vi "HFRR ADV v019 new software.vi"() -> ()   [LabVIEW 2025] (continued)
        n324 = event-data() -> ()  [unwired: 1 in, 6 out]
        n325 = Unbundle By Name("Password 3") -> ("Service Password"=w413:string)
        n326 = call <vilib>:"Trim Whitespace.vi"("string"=w413) -> ("trimmed string"=w411:string)  [unwired: 1 in]
        n327 = Equal?(x=w411, y="Service@123") -> (x = y?=w412:bool)
        n328 = case shown="False" w412 {
          selector: w412 -> [w417 w419]
          frame False {
            n329 = local write "Service Password enable"(w417) -> ()
            n330 = property on="Service Password Log" class="Str"("Visible"=TRUE) -> ()  [unwired: 2 in, 2 out]
            n331 = property on="Tab Control 5" class="TabCtl (strict)"("Tabs Visible?"=TRUE ("Page Labels Display Visible?")) -> ()  [unwired: 2 in, 2 out]
          }
          frame True {
            n332 = property on="Service Password Log" class="Str"("Visible"=FALSE) -> ()  [unwired: 2 in, 2 out]
            "Service Password enable" <- w419
          }
        }
      }
      event "Sign In": Value Change {
        w421 = FALSE ("Visible")
        n333 = event-data() -> ()  [unwired: 1 in, 6 out]
        n334 = property on="About" class="Clust (strict)"("Visible"=w421) -> ()  [unwired: 2 in, 2 out]
        n335 = property on="Password 3" class="Clust (strict)"("Visible"=w421) -> ()  [unwired: 2 in, 2 out]
        n336 = property on="Service Password Log" class="Str"("Visible"=FALSE) -> ()  [unwired: 2 in, 2 out]
      }
      event "Info": Value Change {
        n337 = event-data() -> ()  [unwired: 1 in, 6 out]
        n338 = local read "Info"() -> (w423:bool)
        n339 = case shown="False" w423 {
          frame False {
            n340 = property on="About" class="Clust (strict)"("Visible"=FALSE) -> ()  [unwired: 2 in, 2 out]
          }
          frame True {
            n341 = property on="About" class="Clust (strict)"("Visible"=TRUE) -> ()  [unwired: 2 in, 2 out]
          }
        }
      }
      event "Calibration": Value Change {
        n342 = event-data() -> ()  [unwired: 1 in, 6 out]
        n343 = local read "Calibration"() -> (w427:bool)
        n344 = case shown="False" w427 {
          frame False {
            n345 = property on="Calibration 2" class="TabCtl (strict)"("Visible"=FALSE) -> ()  [unwired: 2 in, 2 out]
            n346 = local write "Cal Password"("" ("Cal Password")) -> ()
          }
          frame True {
            n347 = property on="Calibration 2" class="TabCtl (strict)"("Visible"=TRUE) -> ()  [unwired: 2 in, 2 out]
            n348 = local write "Cal Password"("" ("Cal Password")) -> ()
          }
        }
        n349 = property on="Wrong Password" class="Str"("Visible"=FALSE) -> ()  [unwired: 2 in, 2 out]
      }
      event "Cal Password": Value Change {
        n350 = event-data() -> ()  [unwired: 1 in, 6 out]
        n351 = local read "Cal Password"() -> (w435:string)
        n352 = call <vilib>:"Trim Whitespace.vi"("string"=w435) -> ("trimmed string"=w434:string)  [unwired: 1 in]
        n353 = Equal?(x=w434, y="Cal@321") -> (x = y?=w432:bool)
        n354 = case shown="True" w432 {
          frame False {
            n355 = property on="Wrong Password" class="Str"("Visible"=TRUE) -> ()  [unwired: 2 in, 2 out]
          }
          frame True {
            n356 = property on="Wrong Password" class="Str"("Visible"=FALSE) -> ()  [unwired: 2 in, 2 out]
            n357 = local write "Main Tab"(T2."About" ("Main Tab")) -> ()
            n358 = local write "Cal Password"("" ("Cal Password")) -> ()
            n359 = local write "Main Dashboard Buttons"(T1."About" ("Main Dashboard Buttons")) -> ()
            n360 = local write "Tab Control 5"(T12."Temperature Calibration" ("Tab Control 5")) -> ()
            n361 = property on="Calibration 2" class="TabCtl (strict)"("Visible"=FALSE) -> ()  [unwired: 2 in, 2 out]
            n362 = property on="Tab Control 5" class="TabCtl (strict)"("Tabs Visible?"=FALSE ("Page Labels Display Visible?")) -> ()  [unwired: 2 in, 2 out]
            n363 = local write "Calibration"(FALSE ("Calibration")) -> ()
          }
        }
      }
      event "Calibration Selection": Value Change {
        n364 = event-data() -> ()  [unwired: 1 in, 6 out]
        n365 = local read "Calibration Selection"() -> (w446:T8)
        n366 = case shown="\"Stroke Calibration\"" w446 {
          tunnel: [T7."Stroke" ("Main Calibration Tab") T7."Friction" ("Main Calibration Tab") T7."Main" ("Main Calibration Tab") T7."Temperature" ("Main Calibration Tab")] -> w445
          frame "Stroke Calibration" {
          }
          frame "Friction Force Calibration" {
          }
          frame Default {
          }
          frame "Temperature Calibration" {
          }
        }
        n367 = local write "Main Calibration Tab"(w445) -> ()
      }
      event "Back Stroke": Value Change {
        n368 = event-data() -> ()  [unwired: 1 in, 6 out]
        n369 = local write "Main Stroke Tab"(T9."Step 1" ("Main Stroke Tab")) -> ()
        n370 = local write "Main Calibration Tab"(T7."Main" ("Main Calibration Tab")) -> ()
        n371 = local write "Back Stroke"(FALSE ("Back Stroke")) -> ()
      }
      event "Step 2 Back": Value Change {
        n372 = event-data() -> ()  [unwired: 1 in, 6 out]
        n373 = local write "Main Stroke Tab"(T9."Step 1" ("Main Stroke Tab")) -> ()
        n374 = local write "Step 2 Back"(FALSE ("Back Stroke")) -> ()
      }
      event "Step 3 Back": Value Change {
        n375 = event-data() -> ()  [unwired: 1 in, 6 out]
        n376 = local write "Main Stroke Tab"(T9."Step 2" ("Main Stroke Tab")) -> ()
        n377 = local write "Step 3 Back"(FALSE ("Back Stroke")) -> ()
      }
      event "Step 4 Back": Value Change {
        n378 = event-data() -> ()  [unwired: 1 in, 6 out]
        n379 = local write "Main Stroke Tab"(T9."Step 3" ("Main Stroke Tab")) -> ()
        n380 = local write "Step 4 Back"(FALSE ("Back Stroke")) -> ()
      }
      event "Step 5 Back": Value Change {
        n381 = event-data() -> ()  [unwired: 1 in, 6 out]
        n382 = local write "Main Stroke Tab"(T9."Step 4" ("Main Stroke Tab")) -> ()
        n383 = local write "Step 5 Back"(FALSE ("Back Stroke")) -> ()
      }
      event "Step 6 Back": Value Change {
        n384 = event-data() -> ()  [unwired: 1 in, 6 out]
        n385 = local write "Main Stroke Tab"(T9."Step 5" ("Main Stroke Tab")) -> ()
        n386 = local write "Step 6 Back"(FALSE ("Back Stroke")) -> ()
      }
      event "Back Stroke step 7": Value Change {
        n387 = event-data() -> ()  [unwired: 1 in, 6 out]
        n388 = local write "Main Stroke Tab"(T9."Step 6" ("Main Stroke Tab")) -> ()
        n389 = local write "Back Stroke step 7"(FALSE ("Back Stroke")) -> ()
      }
      event "Back Stroke step 8": Value Change {
        n390 = event-data() -> ()  [unwired: 1 in, 6 out]
        n391 = local write "Main Stroke Tab"(T9."Step 7" ("Main Stroke Tab")) -> ()
        n392 = local write "Back Stroke step 8"(FALSE ("Back Stroke")) -> ()
      }
      event "Back Stroke 8": Value Change {
        n393 = event-data() -> ()  [unwired: 1 in, 6 out]
        n394 = local write "MOVE CARRIAGE TO"(0.2 ("MOVE CARRIAGE TO")) -> ()
        n395 = local write "Main Stroke Tab"(T9."Step 1" ("Main Stroke Tab")) -> ()
        n396 = local write "Back Stroke 8"(FALSE ("Back Stroke 8")) -> ()
      }
      event "Continue Stroke": Value Change {
        n397 = event-data() -> ()  [unwired: 1 in, 6 out]
        n398 = local write "Main Stroke Tab"(T9."Step 2" ("Main Stroke Tab")) -> ()
        n399 = local write "Continue Stroke"(FALSE ("Continue Stroke")) -> ()
      }
      event "Continue Stroke step 2": Value Change {
        n400 = event-data() -> ()  [unwired: 1 in, 6 out]
        n401 = local write "Main Stroke Tab"(T9."Step 3" ("Main Stroke Tab")) -> ()
        n402 = local write "Continue Stroke step 2"(FALSE ("Continue Stroke")) -> ()
      }
      event "Continue Stroke step 3": Value Change {
        n403 = event-data() -> ()  [unwired: 1 in, 6 out]
        n404 = local write "Main Stroke Tab"(T9."Step 4" ("Main Stroke Tab")) -> ()
        n405 = local write "Continue Stroke step 3"(FALSE ("Continue Stroke")) -> ()
      }
      event "Continue Stroke step 4": Value Change {
        n406 = event-data() -> ()  [unwired: 1 in, 6 out]
        n407 = local write "Main Stroke Tab"(T9."Step 5" ("Main Stroke Tab")) -> ()
        n408 = local write "Continue Stroke step 4"(FALSE ("Continue Stroke")) -> ()
      }
      event "Continue Stroke step 5": Value Change {
        n409 = event-data() -> ()  [unwired: 1 in, 6 out]
        n410 = local write "Main Stroke Tab"(T9."Step 6" ("Main Stroke Tab")) -> ()
        n411 = local write "Continue Stroke step 5"(FALSE ("Continue Stroke")) -> ()
      }
      event "Continue Stroke step 6": Value Change {
        n412 = event-data() -> ()  [unwired: 1 in, 6 out]
        n413 = local write "Main Stroke Tab"(T9."Step 7" ("Main Stroke Tab")) -> ()
        n414 = local write "Continue Stroke step 6"(FALSE ("Continue Stroke")) -> ()
      }
      event "Continue Stroke step 7": Value Change {
        w485 = FALSE ("0.2mm")
        n415 = event-data() -> ()  [unwired: 1 in, 6 out]
        n416 = local write "0.4 mm"(w485) -> ()
        n417 = local write "0.6 mm"(w485) -> ()
        n418 = local write "1.0 mm"(w485) -> ()
        n419 = local write "1.2 mm"(w485) -> ()
        n420 = local write "0.2 2"(w485) -> ()
        n421 = local write "0.4 2"(w485) -> ()
        n422 = local write "0.6 2"(w485) -> ()
        n423 = local write "0.8 2"(w485) -> ()
        n424 = local write "1.0 2"(w485) -> ()
        n425 = local write "1.2"(w485) -> ()
        n426 = local write "0.2mm"(w485) -> ()
        n427 = local write "0.8mm"(w485) -> ()
        n428 = local write "Main Stroke Tab"(T9."Step 8" ("Main Stroke Tab")) -> ()
        n429 = local write "Continue Stroke step 7"(FALSE ("Continue Stroke")) -> ()
        n430 = local write "Stroke Test Complete"(T10."Test Progress" ("Stroke Test Complete")) -> ()
        "Position Measurment Temp" <- 0.0 ("Position Measurment Temp")
        "Calibration Tare" <- TRUE ("Calibration Tare")
        "MOVE CARRIAGE TO" <- 0.2 ("MOVE CARRIAGE TO")
      }
      event "Continue Stroke step 8": Value Change {
        n431 = event-data() -> ()  [unwired: 1 in, 6 out]
        n432 = local read "LVDT STROKE  Calibration"() -> (w490:dbl)
        n433 = local read "Position Measurment Temp"() -> (w491:dbl)
        n434 = case shown="4" w491 {
          selector: w491 -> [w496 w501 w506 w511 w516 w520 w523 w524]
          tunnel: w490 -> [w492 w497 w502 w507 w512 w517 _ _]
          frame 0, Default {
            w494 = TRUE ("0.2mm")
            n435 = Increment(x=w496) -> (x+1=w495:i32)
            n436 = local write "Position Measurment Temp"(w495) -> ()
            n437 = local write "0.2mm"(w494) -> ()
            n438 = local write "0.2 2"(w494) -> ()
            n439 = local write "MOVE CARRIAGE TO"(0.4 ("MOVE CARRIAGE TO")) -> ()
            "Calibration 0.2" <- w492
          }
          frame 1 {
            w499 = TRUE ("0.4 mm")
            n440 = Increment(x=w501) -> (x+1=w500:i32)
            n441 = local write "Calibration 0.4"(w497) -> ()
            n442 = local write "Position Measurment Temp"(w500) -> ()
            n443 = local write "0.4 mm"(w499) -> ()
            n444 = local write "MOVE CARRIAGE TO"(0.6 ("MOVE CARRIAGE TO")) -> ()
            n445 = local write "0.4 2"(w499) -> ()
          }
          frame 2 {
            w504 = TRUE ("0.6 mm")
            n446 = Increment(x=w506) -> (x+1=w505:i32)
            n447 = local write "Calibration 0.6"(w502) -> ()
            n448 = local write "Position Measurment Temp"(w505) -> ()
            n449 = local write "0.6 2"(w504) -> ()
            n450 = local write "0.6 mm"(w504) -> ()
            n451 = local write "MOVE CARRIAGE TO"(0.8 ("MOVE CARRIAGE TO")) -> ()
          }
          frame 3 {
            w508 = TRUE ("0.6 mm")
            n452 = Increment(x=w511) -> (x+1=w510:i32)
            n453 = local write "Position Measurment Temp"(w510) -> ()
            n454 = local write "MOVE CARRIAGE TO"(1.0 ("MOVE CARRIAGE TO")) -> ()
            n455 = local write "0.8mm"(w508) -> ()
            n456 = local write "0.8 2"(w508) -> ()
            "Calibration 0.8" <- w507
          }
          frame 4 {
            w513 = TRUE ("0.6 mm")
            n457 = Increment(x=w516) -> (x+1=w515:i32)
            n458 = local write "Position Measurment Temp"(w515) -> ()
            n459 = local write "MOVE CARRIAGE TO"(1.2 ("MOVE CARRIAGE TO")) -> ()
            n460 = local write "1.0 mm"(w513) -> ()
            n461 = local write "1.0 2"(w513) -> ()
            "Calibration 1.0" <- w512
          }
          frame 5 {
            w518 = TRUE ("0.6 mm")
            n462 = Increment(x=w520) -> (x+1=w519:i32)
            n463 = local write "Position Measurment Temp"(w519) -> ()
            n464 = local write "1.2 mm"(w518) -> ()
            n465 = local write "1.2"(w518) -> ()
            "Calibration 1.2" <- w517
          }
          frame 6 {
            n466 = Increment(x=w523) -> (x+1=w522:i32)
            n467 = local write "Position Measurment Temp"(w522) -> ()
            n468 = local write "Stroke Test Complete"(T10."Stroke Points Completed" ("Stroke Test Complete")) -> ()
          }
          frame 7 {
            n469 = stacked-sequence {
              tunnel: w524 -> [w525 _ _]
              frame #0 {
                n470 = Increment(x=w525) -> (x+1=w526:i32)
                n471 = local write "Main Stroke Tab"(T9."Step 9" ("Main Stroke Tab")) -> ()
                n472 = local write "Position Measurment Temp"(w526) -> ()
                n473 = Insert Into Array(array=dbl[] [], new element #1=0.2 ("new element/subarray"), new element #2=0.4 ("new element/subarray"), new element #3=0.6 ("new element/subarray"), new element #4=0.8 ("new element/subarray"), new element #5=1.0 ("new element/subarray"), new element #6=1.2 ("new element/subarray")) -> (→"1D stroke":dbl[])  [unwired: 1 in]
                n474 = local read "Calibration 0.2"() -> (w533:dbl)
                n475 = local read "Calibration 0.4"() -> (w532:dbl)
                n476 = local read "Calibration 0.6"() -> (w531:dbl)
                n477 = local read "Calibration 0.8"() -> (w530:dbl)
                n478 = local read "Calibration 1.0"() -> (w529:dbl)
                n479 = local read "Calibration 1.2"() -> (w528:dbl)
                n480 = Insert Into Array(array=dbl[] [], new element #1=w533, new element #2=w532, new element #3=w531, new element #4=w530, new element #5=w529, new element #6=w528) -> (→"Calibrated Voltage Value":dbl[])  [unwired: 1 in]
              }
              frame #1 {
                n481 = local read "Calibrated Voltage Value"() -> (w545:dbl[])
                n482 = local read "1D stroke"() -> (w546:dbl[])
                n483 = for {
                  tunnel: [w549] -> w544 mode=indexing
                  tunnel: w546 -> [w548] mode=indexing
                  tunnel: w545 -> [w547] mode=indexing
                  n484 = formula code="if (stroke == 0.2) {\n    status = (voltage >= 0.0961 && voltage <= 0.4961) ? 1 : 0;\n} else if (stroke == 0.4) {\n    status = (voltage >= 0.3425 && voltage <= 0.7425) ? 1 : 0;\n} else if (stroke == 0.6) {\n    status = (voltage >= 0.5370 && voltage <= 0.9370) ? 1 : 0;\n} else if (stroke == 0.8) {\n    status = (voltage >= 0.6640 && voltage <= 1.0640) ? 1 : 0;\n} else if (stroke == 1.0) {\n    status = (voltage >= 0.9000 && voltage <= 1.1000) ? 1 : 0;\n} else if (stroke == 1.2) {\n    status = (voltage >= 0.9278 && voltage <= 1.3278) ? 1 : 0;\n} else {\n    status = 0; // Fails if an invalid stroke value is supplied\n}"("stroke"=w548, "voltage"=w547) -> ("status"=w549:dbl)
                }
                "Status" <- w544
              }
              frame #2 {
                w556 = 1.0
                n485 = local read "Status"() -> (w563:dbl[])
                n486 = Index Array(array=w563) -> (element #1=w562:dbl, element #2=w561:dbl, element #3=w560:dbl, element #4=w559:dbl, element #5=w558:dbl, element #6=w557:dbl)  [unwired: 6 in]
                n487 = Equal?(x=w561, y=w556) -> (x = y?=w554:bool)
                n488 = Equal?(x=w560, y=w556) -> (x = y?=w553:bool)
                n489 = Equal?(x=w559, y=w556) -> (x = y?=w552:bool)
                n490 = Equal?(x=w558, y=w556) -> (x = y?=w551:bool)
                n491 = Equal?(x=w557, y=w556) -> (x = y?=w550:bool)
                n492 = Equal?(x=w562, y=w556) -> (x = y?=w555:bool)
                n493 = case shown="True" w555 {
                  selector: w555 -> [w574 w575]
                  frame True {
                    n494 = local write "Point 1 - 0.2 mm"(w574) -> ()
                    n495 = property on="Point 1 - 0.2 mm" class="Bool"("Caption.Visible"=w574) -> ()  [unwired: 2 in, 2 out]
                  }
                  frame False {
                    n496 = local write "Point 1 - 0.2 mm"(w575) -> ()
                    n497 = property on="Point 1 - 0.2 mm" class="Bool"("Caption.Visible"=w575) -> ()  [unwired: 2 in, 2 out]
                  }
                }
                n498 = case shown="True" w554 {
                  selector: w554 -> [w572 w573]
                  frame True {
                    n499 = local write "Point 2 - 0.4 mm"(w572) -> ()
                    n500 = property on="Point 2 - 0.4 mm" class="Bool"("Caption.Visible"=w572) -> ()  [unwired: 2 in, 2 out]
                  }
                  frame False {
                    n501 = local write "Point 2 - 0.4 mm"(w573) -> ()
                    n502 = property on="Point 2 - 0.4 mm" class="Bool"("Caption.Visible"=w573) -> ()  [unwired: 2 in, 2 out]
                  }
                }
                n503 = case shown="True" w551 {
                  selector: w551 -> [w566 w567]
                  frame True {
                    n504 = local write "Point 5 - 1.0 mm"(w566) -> ()
                    n505 = property on="Point 5 - 1.0 mm" class="Bool"("Caption.Visible"=w566) -> ()  [unwired: 2 in, 2 out]
                  }
                  frame False {
                    n506 = local write "Point 5 - 1.0 mm"(w567) -> ()
                    n507 = property on="Point 5 - 1.0 mm" class="Bool"("Caption.Visible"=w567) -> ()  [unwired: 2 in, 2 out]
                  }
                }
                n508 = case shown="True" w553 {
                  selector: w553 -> [w570 w571]
                  frame True {
                    n509 = local write "Point 3 - 0.6 mm"(w570) -> ()
                    n510 = property on="Point 3 - 0.6 mm" class="Bool"("Caption.Visible"=w570) -> ()  [unwired: 2 in, 2 out]
                  }
                  frame False {
                    n511 = local write "Point 3 - 0.6 mm"(w571) -> ()
                    n512 = property on="Point 3 - 0.6 mm" class="Bool"("Caption.Visible"=w571) -> ()  [unwired: 2 in, 2 out]
                  }
                }
                n513 = case shown="True" w552 {
                  selector: w552 -> [w568 w569]
                  frame True {
                    n514 = local write "Point 4 - 0.8 mm"(w568) -> ()
                    n515 = property on="Point 4 - 0.8 mm" class="Bool"("Caption.Visible"=w568) -> ()  [unwired: 2 in, 2 out]
                  }
                  frame False {
                    n516 = local write "Point 4 - 0.8 mm"(w569) -> ()
                    n517 = property on="Point 4 - 0.8 mm" class="Bool"("Caption.Visible"=w569) -> ()  [unwired: 2 in, 2 out]
                  }
                }
                n518 = case shown="True" w550 {
                  selector: w550 -> [w564 w565]
                  frame True {
                    n519 = local write "Point 6 - 1.2 mm"(w564) -> ()
                    n520 = property on="Point 6 - 1.2 mm" class="Bool"("Caption.Visible"=w564) -> ()  [unwired: 2 in, 2 out]
                  }
                  frame False {
                    n521 = local write "Point 6 - 1.2 mm"(w565) -> ()
                    n522 = property on="Point 6 - 1.2 mm" class="Bool"("Caption.Visible"=w565) -> ()  [unwired: 2 in, 2 out]
                  }
                }
              }
            }
          }
        }
      }
      event "TEMPERATURE STEP Back 1", "TEMPERATURE STEP Back air Temp": Value Change {
        n523 = event-data() -> ()  [unwired: 1 in, 6 out]
        n524 = stacked-sequence {
          frame #0 {
            n525 = local write "Main Calibration Tab"(T7."Main" ("Main Calibration Tab")) -> ()
          }
          frame #1 {
            n526 = Wait (ms)(milliseconds to wait=u32 1000) -> ()  [unwired: 1 out]
          }
          frame #2 {
            n527 = local write "Command"("CAL;END" ("Command")) -> ()
          }
          frame #3 {
            n528 = Wait (ms)(milliseconds to wait=u32 2000) -> ()  [unwired: 1 out]
          }
          frame #4 {
            n529 = local write "Command"("CAL;END" ("Command")) -> ()
          }
        }
      }
      event "Temperature Continue Step 1": Value Change {
        n530 = event-data() -> ()  [unwired: 1 in, 6 out]
        n531 = stacked-sequence {
          frame #0 {
            n532 = Wait (ms)(milliseconds to wait=u32 1500) -> ()  [unwired: 1 out]
          }
          frame #1 {
            n533 = local write "Command"("CAL;START" ("Command")) -> ()
          }
          frame #2 {
            n534 = Wait (ms)(milliseconds to wait=u32 1500) -> ()  [unwired: 1 out]
          }
          frame #3 {
            n535 = local write "Command"("CAL;START" ("Command")) -> ()
          }
          frame #4 {
            n536 = Wait (ms)(milliseconds to wait=u32 2000) -> ()  [unwired: 1 out]
          }
          frame #5 {
          }
          frame #6 {
            n537 = Wait (ms)(milliseconds to wait=u32 2000) -> ()  [unwired: 1 out]
          }
          frame #7 {
            # "CAL;A1;<true_T>"
            n538 = local write "Command"("CAL;A1;0" ("Command")) -> ()
          }
          frame #8 {
            n539 = local write "Tab Control 4"(T11."Step 2" ("Tab Control 4")) -> ()
          }
        }
      }
      event "Temperature Continue Step air Step 1": Value Change {
        n540 = event-data() -> ()  [unwired: 1 in, 6 out]
        n541 = stacked-sequence {
          frame #0 {
            n542 = Wait (ms)(milliseconds to wait=u32 1500) -> ()  [unwired: 1 out]
          }
          frame #1 {
            n543 = local write "Command"("CAL;START" ("Command")) -> ()
          }
          frame #2 {
            n544 = local write "Tab Control 4"(T11."Air Step 2" ("Tab Control 4")) -> ()
            n545 = Wait (ms)(milliseconds to wait=u32 1500) -> ()  [unwired: 1 out]
          }
          frame #3 {
            n546 = local write "Command"("CAL;START" ("Command")) -> ()
          }
          frame #4 {
            n547 = Wait (ms)(milliseconds to wait=u32 2000) -> ()  [unwired: 1 out]
          }
          frame #5 {
            # "CAL;A1;<true_T>"
            n548 = local write "Command"("CAL;A2;0" ("Command")) -> ()
          }
          frame #6 {
            n549 = Wait (ms)(milliseconds to wait=u32 2000) -> ()  [unwired: 1 out]
          }
          frame #7 {
            # "CAL;A1;<true_T>"
            n550 = local write "Command"("CAL;A1;0" ("Command")) -> ()
          }
        }
      }
      event "Temperature Selection": Value Change {
        n551 = event-data() -> ()  [unwired: 1 in, 6 out]
        n552 = local read "Temperature Selection"() -> (w598:enum32{"Air Temperature", "Sample Temperature"})
        n553 = case shown="\"Sample Temperature\"" w598 {
          frame "Air Temperature", Default {
            n554 = local write "Tab Control 4"(T11."Air Step 1" ("Tab Control 4")) -> ()
          }
          frame "Sample Temperature" {
            n555 = local write "Tab Control 4"(T11."Step 1" ("Tab Control 4")) -> ()
          }
        }
      }
      event "Temperature Continue Step 2": Value Change {
        n556 = event-data() -> ()  [unwired: 1 in, 6 out]
        n557 = stacked-sequence {
          frame #0 {
            n558 = stacked-sequence {
              frame #0 {
                n559 = Wait (ms)(milliseconds to wait=u32 1500) -> ()  [unwired: 1 out]
              }
              frame #1 {
                # "CAL;A1;<true_T>"
                n560 = local write "Command"("CAL;A1;0" ("Command")) -> ()
              }
              frame #2 {
                n561 = Wait (ms)(milliseconds to wait=u32 1500) -> ()  [unwired: 1 out]
              }
              frame #3 {
                # "CAL;A1;<true_T>"
                n562 = local write "Command"("CAL;A1;0" ("Command")) -> ()
              }
              frame #4 {
              }
            }
          }
          frame #1 {
            n563 = local write "Tab Control 4"(T11."Step 3" ("Tab Control 4")) -> ()
          }
        }
      }
      event "Temperature Continue Step 3": Value Change {
        n564 = event-data() -> ()  [unwired: 1 in, 6 out]
        n565 = stacked-sequence {
          frame #0 {
            n566 = stacked-sequence {
              frame #0 {
                n567 = Wait (ms)(milliseconds to wait=u32 1500) -> ()  [unwired: 1 out]
              }
              frame #1 {
              }
              frame #2 {
              }
              frame #3 {
                # "CAL;A1;<true_T>"
                n568 = local write "Command"("CAL;A1;60" ("Command")) -> ()
              }
              frame #4 {
                n569 = Wait (ms)(milliseconds to wait=u32 2000) -> ()  [unwired: 1 out]
              }
              frame #5 {
                # "CAL;A1;<true_T>"
                n570 = local write "Command"("CAL;A1;60" ("Command")) -> ()
              }
            }
          }
          frame #1 {
            n571 = Wait (ms)(milliseconds to wait=u32 1000) -> ()  [unwired: 1 out]
          }
          frame #2 {
            n572 = local write "Command"("CAL;SAVE" ("Command")) -> ()
          }
          frame #3 {
            n573 = Wait (ms)(milliseconds to wait=u32 1000) -> ()  [unwired: 1 out]
          }
          frame #4 {
            n574 = local write "Command"("CAL;SAVE" ("Command")) -> ()
          }
          frame #5 {
            n575 = Wait (ms)(milliseconds to wait=u32 1000) -> ()  [unwired: 1 out]
          }
          frame #6 {
            # "CAL;END"
            n576 = local write "Command"("CAL;END" ("Command")) -> ()
          }
          frame #7 {
            n577 = Wait (ms)(milliseconds to wait=u32 1000) -> ()  [unwired: 1 out]
          }
          frame #8 {
            # "CAL;END"
            n578 = local write "Command"("CAL;END" ("Command")) -> ()
          }
          frame #9 {
            n579 = local write "Main Calibration Tab"(T7."Temperature" ("Main Calibration Tab")) -> ()
            n580 = local write "Tab Control 4"(T11."Main" ("Tab Control 4")) -> ()
          }
        }
      }
      event "Back Stroke step main temperature": Value Change {
        n581 = event-data() -> ()  [unwired: 1 in, 6 out]
        n582 = stacked-sequence {
          frame #0 {
            n583 = Wait (ms)(milliseconds to wait=u32 1000) -> ()  [unwired: 1 out]
          }
          frame #1 {
            # "CAL;END"
            n584 = local write "Command"("CAL;END" ("Command")) -> ()
          }
          frame #2 {
            n585 = Wait (ms)(milliseconds to wait=u32 1000) -> ()  [unwired: 1 out]
          }
          frame #3 {
            # "CAL;END"
            n586 = local write "Command"("CAL;END" ("Command")) -> ()
          }
          frame #4 {
            n587 = local write "Main Calibration Tab"(T7."Temperature" ("Main Calibration Tab")) -> ()
            n588 = local write "Tab Control 4"(T11."Main" ("Tab Control 4")) -> ()
          }
        }
      }
      event "Quit": Value Change {
        n589 = event-data() -> ()  [unwired: 1 in, 6 out]
      }
    }
    n590 = Wait (ms)(milliseconds to wait=u32 100) -> ()  [unwired: 1 out]
  }
  n591 = while {
    stop <- w630 stop-if-true
    n592 = local read "Ambient Temperature"() -> (w628:dbl)
    n593 = local read "Sample Temperature"() -> (w627:dbl)
    n594 = local write "Temperature — Live (Set A: 60 °C)"(w627) -> ()
    n595 = local write "Temperature — Live (Set A: 60 °C)"(w627) -> ()
    n596 = local write "Temperature — Live (Set A: 0 °C)"(w628) -> ()
    n597 = local write "Sensor value"(w628) -> ()
    n598 = local write "Sensor value"(w627) -> ()
    n599 = local write "Temperature — Live (Set A: 60 °C)"(w628) -> ()
    n600 = local write "Sensor value"(w627) -> ()
    n601 = local write "Sensor value"(w628) -> ()
    n602 = Wait (ms)(milliseconds to wait=u32 200) -> ()  [unwired: 1 out]
    n603 = local read "Quit"() -> (w630:bool)
  }
  n604 = while {
    shift-right: [w632] -> _
    shift-left: "Enum - Selector" -> [w633]
    stop <- w634 stop-if-true
    # "Auto Start Logic Loop"
    n605 = case shown="\"Humidity & Temperature On\"" w633 {
      tunnel: [w637 w643 w670 w702 w732 Auto_Start_enum."Exit" ("Enum - Selector") Auto_Start_enum."Init" ("Enum - Selector")] -> w632
      frame "Init", Default {
        n606 = local read "Auto Start Test"() -> (w636:bool)
        n607 = Select(t=Auto_Start_enum."Humidity & Temperature On" ("Enum - Selector"), s=w636, f=Auto_Start_enum."Init") -> (s? t:f=w637:T15)
      }
      frame "Humidity & Temperature On" {
        n608 = stacked-sequence {
          tunnel: [_ _ _ _ _ _ Auto_Start_enum."Reach point" ("Enum - Selector")] -> w640
          frame #0 {
            w645 = T19."Disabled and Grayed Out" ("Disabled")
            w646 = TRUE ("Heater Button")
            n609 = property on="Humidity" class="Bool (strict)"("DisabledEnum"=w645) -> ()  [unwired: 2 in, 2 out]
            n610 = property on="Heater Button" class="Bool (strict)"("DisabledEnum"=w645) -> ()  [unwired: 2 in, 2 out]
            n611 = local write "Heater Button"(w646) -> ()
            n612 = local write "Humidity"(w646) -> ()
            n613 = property on="Heater Button" class="Bool (strict)"("Val(Sgnl)"=TRUE ("Value (Signaling)")) -> ()  [unwired: 2 in, 2 out]
          }
          frame #1 {
            n614 = Wait (ms)(milliseconds to wait=u32 3000) -> ()  [unwired: 1 out]
          }
          frame #2 {
            n615 = local read "Set Temp"() -> (w652:dbl)
            n616 = Number To Fractional String(number=w652, precision (6)=i16 2) -> (F-format string=w649:string)  [unwired: 2 in]
            n617 = Concatenate Strings("ST;" ("Command"), w649) -> (w650:string)
            n618 = local write "Command"(w650) -> ()
          }
          frame #3 {
            n619 = Wait (ms)(milliseconds to wait=u32 1500) -> ()  [unwired: 1 out]
          }
          frame #4 {
            (unwired) i16 2 ("precision (6)")
            n620 = local read "WriteHumidity 2"() -> (w654:string[])
            n621 = local read "Set Rh"() -> (w657:dbl)
            n622 = Number To Fractional String(number=w657) -> (F-format string=w658:string)  [unwired: 3 in]
            n623 = Concatenate Strings("M;" ("new element/subarray"), w658) -> (w659:string)
            n624 = local write "Command"("HE;1" ("Command")) -> ()
            n625 = Insert Into Array(array=w654, new element=w659) -> (w655:string[])  [unwired: 1 in]
            n626 = local write "WriteHumidity 2"(w655) -> ()
          }
          frame #5 {
            n627 = Wait (ms)(milliseconds to wait=u32 1500) -> ()  [unwired: 1 out]
          }
          frame #6 {
            w662 = TRUE ("Reach point temp")
            n628 = local write "Reach point Humidity"(w662) -> ()
            n629 = local write "Reach point temp"(w662) -> ()
          }
        }
        n630 = local read "Auto Start Test"() -> (w642:bool)
        n631 = Not(x=w642) -> (.not. x?=w641:bool)
        n632 = Select(t=Auto_Start_enum."close", s=w641, f=w640) -> (s? t:f=w643:T15)
      }
      frame "Reach point" {
        w671 = TRUE ("PAUSE")
        w679 = 1.0 ("y")
        w682 = 1.0 ("y")
        n633 = local read "Set Temp"() -> (w664:dbl)
        n634 = local read "Set Humidity:"() -> (w678:dbl)
        n635 = local read "Humidity ( %RH )"() -> (w683:dbl)
        n636 = Add(x=w664, y=w682) -> (x+y=w681:dbl)
        n637 = Subtract(x=w664, y=w682) -> (x-y=w680:dbl)
        n638 = Add(x=w678, y=w679) -> (x+y=w677:dbl)
        n639 = Subtract(x=w678, y=w679) -> (x-y=w676:dbl)
        n640 = local read "TEMP"() -> (w684:dbl)
        n641 = In Range and Coerce(upper limit=w677, x=w683, lower limit=w676) -> (In Range?=w665:bool)  [unwired: 1 out]
        n642 = In Range and Coerce(upper limit=w681, x=w684, lower limit=w680) -> (In Range?=w666:bool)  [unwired: 1 out]
        n643 = case shown="True" w665 {
          frame False {
          }
          frame True {
            n644 = case shown="True" "Reach point Humidity" {
              selector: "Reach point Humidity" -> [_ w690]
              frame False {
              }
              frame True {
                n645 = local read "EVENT LOG"() -> (w687:string)
                n646 = Not(x=w690) -> (.not. x?=w689:bool)
                n647 = local write "Reach point Humidity"(w689) -> ()
                n648 = call "Event Log.vi"("Content"="Target Humidity reached", "EVENT LOG"=w687) -> ("EVENT LOG"=w688:string)  [unwired: 8 in, 1 out]
                n649 = local write "EVENT LOG"(w688) -> ()
              }
            }
          }
        }
        n650 = case shown="True" w666 {
          frame False {
          }
          frame True {
            n651 = case shown="True" "Reach point temp" {
              selector: "Reach point temp" -> [_ w696]
              frame False {
              }
              frame True {
                n652 = local read "EVENT LOG"() -> (w693:string)
                n653 = Not(x=w696) -> (.not. x?=w695:bool)
                n654 = local write "Reach point temp"(w695) -> ()
                n655 = call "Event Log.vi"("Content"="Target Temperature reached", "EVENT LOG"=w693) -> ("EVENT LOG"=w694:string)  [unwired: 8 in, 1 out]
                n656 = local write "EVENT LOG"(w694) -> ()
              }
            }
          }
        }
        n657 = local read "Auto Start Test"() -> (w669:bool)
        n658 = And(x=w666, y=w665) -> (x .and. y?=w675:bool)
        n659 = Select(t=Auto_Start_enum."Maintain Stage" ("Enum - Selector"), s=w675, f=Auto_Start_enum."Reach point" ("Enum - Selector")) -> (s? t:f=w672:T15)
        n660 = Not(x=w669) -> (.not. x?=w668:bool)
        n661 = Select(t=Auto_Start_enum."close", s=w668, f=w672) -> (s? t:f=w670:T15)
        n662 = call "ELAPSED TIMER VI.vi"("RESET"=w671, "PAUSE"=w671) -> ()  [unwired: 7 in, 3 out]
      }
      frame "Maintain Stage" {
        w711 = 2.0 ("y")
        w710 = 1.0 ("y")
        # "Humidity and  temperatures Set Point  have been reached"
        n663 = local read "Set Temp"() -> (w697:dbl)
        n664 = local read "Set Humidity:"() -> (w714:dbl)
        n665 = local read "Humidity ( %RH )"() -> (w717:dbl)
        n666 = Add(x=w697, y=w710) -> (x+y=w716:dbl)
        n667 = Subtract(x=w697, y=w710) -> (x-y=w715:dbl)
        n668 = local read "TEMP"() -> (w718:dbl)
        n669 = Add(x=w714, y=w711) -> (x+y=w713:dbl)
        n670 = Subtract(x=w714, y=w711) -> (x-y=w712:dbl)
        n671 = In Range and Coerce(upper limit=w716, x=w718, lower limit=w715) -> (In Range?=w709:bool)  [unwired: 1 out]
        n672 = In Range and Coerce(upper limit=w713, x=w717, lower limit=w712) -> (In Range?=w708:bool)  [unwired: 1 out]
        n673 = And(x=w709, y=w708) -> (x .and. y?=w707:bool)
        n674 = Not(x=w707) -> (.not. x?=w706:bool)
        n675 = call "ELAPSED TIMER VI.vi"("TARGET"=60.0, "RESET"=w706, "PAUSE"=FALSE) -> ("ELAPSED INDICATION"=w703:bool)  [unwired: 6 in, 2 out]
        n676 = case shown="True" w703 {
          tunnel: w703 -> [_ w721]
          tunnel: [Auto_Start_enum."Maintain Stage" ("Enum - Selector") w720] -> w701
          frame False {
          }
          frame True {
            n677 = stacked-sequence {
              tunnel: w721 -> [_ _ _ _ _]
              tunnel: [_ _ _ _ Auto_Start_enum."Start Stage" ("Enum - Selector")] -> w720
              frame #0 {
                n678 = local read "EVENT LOG"() -> (w723:string)
                n679 = call "Event Log.vi"("Content"="Humidity and temperature set point has stabilized.", "EVENT LOG"=w723) -> ("EVENT LOG"=w724:string)  [unwired: 8 in, 1 out]
                n680 = local write "EVENT LOG"(w724) -> ()
              }
              frame #1 {
                n681 = Wait (ms)(milliseconds to wait=u32 100) -> ()  [unwired: 1 out]
              }
              frame #2 {
                n682 = local read "EVENT LOG"() -> (w727:string)
                n683 = call "Event Log.vi"("Content"="Auto Test Started", "EVENT LOG"=w727) -> ("EVENT LOG"=w728:string)  [unwired: 8 in, 1 out]
                n684 = local write "EVENT LOG"(w728) -> ()
              }
              frame #3 {
                w729 = TRUE ("RUN")
                n685 = local write "RUN"(w729) -> ()
                n686 = property on="Auto Start Temp" class="Bool (strict)"("Val(Sgnl)"=w729) -> ()  [unwired: 2 in, 2 out]
                "Auto Start Temp" <- w729
              }
              frame #4 {
              }
            }
          }
        }
        n687 = local read "Auto Start Test"() -> (w700:bool)
        n688 = Not(x=w700) -> (.not. x?=w699:bool)
        n689 = Select(t=Auto_Start_enum."close", s=w699, f=w701) -> (s? t:f=w702:T15)
      }
      frame "Start Stage" {
        w731 = TRUE ("PAUSE")
        n690 = local read "Auto Start Test"() -> (w736:bool)
        n691 = Not(x=w736) -> (.not. x?=w735:bool)
        n692 = Select(t=Auto_Start_enum."close" ("Enum - Selector"), s=w735, f=Auto_Start_enum."Start Stage" ("Enum - Selector")) -> (s? t:f=w732:T15)
        n693 = call "ELAPSED TIMER VI.vi"("RESET"=w731, "PAUSE"=w731) -> ()  [unwired: 7 in, 3 out]
      }
      frame "close" {
        w738 = FALSE ("Heater Button")
        n694 = local write "RUN"(w738) -> ()
        n695 = local write "Heater Button"(w738) -> ()
        n696 = local write "Humidity"(w738) -> ()
        n697 = local write "Auto Start Test"(w738) -> ()
        n698 = property on="Heater Button" class="Bool (strict)"("Val(Sgnl)"=FALSE ("Value (Signaling)")) -> ()  [unwired: 2 in, 2 out]
      }
      frame "Exit" {
      }
    }
    n699 = Wait (ms)(milliseconds to wait=u32 100) -> ()  [unwired: 1 out]
    n700 = local read "Quit"() -> (w634:bool)
  }
  n701 = property on="Service Password Log" class="Str"("Visible"=w16) -> ()  [unwired: 2 in, 2 out]
  n702 = property on="Password 3" class="Clust (strict)"("Visible"=w16) -> ()  [unwired: 2 in, 2 out]
  n703 = while {
    stop <- w767 stop-if-true
    w750 = errorcluster {"status"=FALSE, "code"=0, "source"=""} ("error in (no error) 3")
    # "this loop is for manual report generation"
    n704 = local read "Confirm Measrurement"() -> (w749:bool)
    n705 = case shown="True" w749 {
      selector: w749 -> [_ w857]
      tunnel: errorcluster {"status"=FALSE, "code"=0, "source"=""} ("error in (no error) 3") -> [_ w858]
      tunnel: [_ w856] -> _
      frame False {
      }
      frame True {
        n706 = stacked-sequence {
          tunnel: w858 -> [_ w891 _]
          tunnel: w857 -> [_ _ w998]
          tunnel: [_ w879 _] -> w856
          frame #0 {
            n707 = String To Path(string="C:\\LAB-IQ\\Image Calibrate v01.dcf") -> (path=w861:path)
            n708 = Open/Create/Replace File ("Open File")(file path (use dialog)=w861) -> (refnum out=w862:refnum<file>)  [unwired: 5 in, 2 out]
            n709 = for {
              N: 4 -> [_]
              tunnel: w862 -> [w868]
              i -> [w864]
              n710 = Read from Text File ("Read File")(file (use dialog)=w868) -> (text=w869:string)  [unwired: 3 in, 3 out]
              n711 = String Subset(string=w869, offset (0)=6, length (rest)=10 ("length (rest)")) -> (substring=w865:string)
              n712 = Fract/Exp String To Number(string=w865) -> (number=w863:dbl)  [unwired: 3 in, 1 out]
              n713 = case shown="3" w864 {
                tunnel: w863 -> [w870 w871 _ w872 _]
                frame 0 {
                  n714 = local write "5x Gain"(w870) -> ()
                }
                frame 1 {
                  n715 = local write "10x Gain"(w871) -> ()
                }
                frame 2 {
                }
                frame 3 {
                  n716 = local write "100x gain"(w872) -> ()
                }
                frame 4, Default {
                }
              }
            }
          }
          frame #1 {
            n717 = local read "TEST STANDARD"() -> (w874:T3)
            n718 = case shown="\"ISO 12156\"" w874 {
              tunnel: ["ASTM D6079" "ISO 12156"] -> w873
              frame "ASTM D6079", Default {
              }
              frame "ISO 12156" {
              }
            }
            n719 = call "IMAGE ANALYSIS.vi"("Enum"=POST_ANALYSIS_ENUM."GET MEASUREMENTS", "error in"=w891) -> ("error out"=w898:errorcluster)  [unwired: 8 in, 1 out]
            n720 = local read "Magnification :"() -> (w884:string)
            n721 = call "Stall Data Flow.vim"("value in"=w898, "milliseconds to wait"=u32 1000) -> ("value out"=w897:errorcluster)  [unwired: 1 out]
            n722 = local read "Test File List :"() -> (w895:string)
            n723 = case shown="\"10x\"" w884 {
              tunnel: [w934 w935] -> w882
              frame "5x", Default {
                n724 = local read "5x Gain"() -> (w934:dbl)
              }
              frame "10x" {
                # "5x"
                n725 = local read "10x Gain"() -> (w935:dbl)
              }
            }
            n726 = call "IMAGE ANALYSIS.vi"("Enum"=POST_ANALYSIS_ENUM."READ", "error in"=w897) -> ("error out"=w894:errorcluster, "data out"=w885:string)  [unwired: 8 in]
            n727 = Match Pattern(string=w885, regular expression="\"type\": ") -> (after substring=w889:string)  [unwired: 1 in, 3 out]
            n728 = call "IMAGE PATH CREATION PY.vi"("error in (no error)"=w894, "File Name :"=w895) -> ("error out"=w893:errorcluster, "File Path"=w881:path, "File Path String:"=w876:string)  [unwired: 7 in]
            n729 = Match Pattern(string=w889, regular expression=",") -> (before substring=w875:string)  [unwired: 1 in, 3 out]
            n730 = local read "Calibration Tab"() -> (w878:enum32{"Measrument", "Calibrate"})
            n731 = call "Stall Data Flow.vim"("value in"=w893, "milliseconds to wait"=u32 250) -> ("value out"=w877:errorcluster)  [unwired: 1 out]
            n732 = Equal?(x=w875, y="\"rectangle\"") -> (x = y?=w886:bool)
            n733 = case shown="False" w886 {
              tunnel: w885 -> [w940 w995]
              tunnel: w882 -> [_ w986]
              tunnel: cluster{"major":dbl, "minor":dbl, "average":dbl} {"major"=0.0, "minor"=0.0, "average"=0.0} -> [w938 w982]
              tunnel: [w937 w979] -> w880
              tunnel: w875 -> [w939 _]
              tunnel: w882 -> [w936 _]
              frame False {
                n734 = Equal?(x=w939, y="\"line\"") -> (x = y?=w941:bool)
                n735 = case shown="True" w941 {
                  tunnel: w940 -> [_ w956]
                  tunnel: w938 -> [w943 w955]
                  tunnel: [w943 w953] -> w937
                  tunnel: w936 -> [_ w952]
                  frame False {
                  }
                  frame True {
                    w951 = 0.0 ("Major Axis")
                    n736 = Match Pattern(string=w956, regular expression="\"length_px\":") -> (after substring=w954:string)  [unwired: 1 in, 3 out]
                    n737 = property on="Major Axis" class="DigNum (strict)"("Caption.Text"="") -> ()  [unwired: 2 in, 2 out]
                    n738 = property on="Minor Axis" class="DigNum (strict)"("Caption.Text"="") -> ()  [unwired: 2 in, 2 out]
                    n739 = property on="Average" class="DigNum (strict)"("Caption.Text"="Line") -> ()  [unwired: 2 in, 2 out]
                    n740 = Fract/Exp String To Number(string=w954, default (0 dbl)=0.0 ("default (0 DBL)")) -> (number=w950:dbl)  [unwired: 2 in, 1 out]
                    "Pixel Value" <- w950
                    n741 = Multiply(x=w950, y=w952) -> (x*y=w963:dbl)
                    n742 = Multiply(x=w963, y=1000.0) -> (x*y=w946:dbl)
                    n743 = Divide(x=w946, y=1000.0) -> (x/y=w949:dbl)
                    n744 = local write "Measurment (mm)"(w949) -> ()
                    n745 = Bundle By Name(cluster=w955, "average"=w946) -> (w953:cluster{"major":dbl, "minor":dbl, "average":dbl})
                    n746 = Number To Fractional String(number=w946, precision (6)=i16 1) -> (F-format string=w945:string)  [unwired: 2 in]
                    n747 = local write "Minor Axis"(w951) -> ()
                    n748 = local write "Major Axis"(w951) -> ()
                    n749 = Fract/Exp String To Number(string=w945) -> (number=w944:dbl)  [unwired: 3 in, 1 out]
                    n750 = local write "Average"(w944) -> ()
                  }
                }
              }
              frame True {
                w983 = 1000.0 ("y")
                w989 = 0.0 ("default (0 DBL)")
                n751 = Match Pattern(string=w995, regular expression=" \"width_px\":") -> (after substring=w993:string)  [unwired: 1 in, 3 out]
                n752 = Match Pattern(string=w993, regular expression="\"height_px\":") -> (before substring=w991:string, after substring=w990:string)  [unwired: 1 in, 2 out]
                n753 = Fract/Exp String To Number(string=w991, default (0 dbl)=w989) -> (number=w988:dbl)  [unwired: 2 in, 1 out]
                n754 = Fract/Exp String To Number(string=w990, default (0 dbl)=w989) -> (number=w987:dbl)  [unwired: 2 in, 1 out]
                n755 = Multiply(x=w988, y=w986) -> (x*y=w985:dbl)
                n756 = Multiply(x=w987, y=w986) -> (x*y=w984:dbl)
                n757 = Multiply(x=w985, y=w983) -> (x*y=w969:dbl)
                n758 = Multiply(x=w984, y=w983) -> (x*y=w967:dbl)
                n759 = Add(x=w969, y=w967) -> (x+y=w981:dbl)
                n760 = property on="Major Axis" class="DigNum (strict)"("Caption.Text"="Major Axis") -> ()  [unwired: 2 in, 2 out]
                n761 = property on="Minor Axis" class="DigNum (strict)"("Caption.Text"="Minor Axis") -> ()  [unwired: 2 in, 2 out]
                n762 = property on="Average" class="DigNum (strict)"("Caption.Text"="Average") -> ()  [unwired: 2 in, 2 out]
                n763 = Divide(x=w981, y=2.0) -> (x/y=w965:dbl)
                n764 = Bundle By Name(cluster=w982, "major"=w969, "minor"=w967, "average"=w965) -> (w979:cluster{"major":dbl, "minor":dbl, "average":dbl})
                n765 = Number To Fractional String(number=w967, precision (6)=i16 1) -> (F-format string=w974:string)  [unwired: 2 in]
                n766 = Number To Fractional String(number=w965, precision (6)=i16 1) -> (F-format string=w975:string)  [unwired: 2 in]
                n767 = Number To Fractional String(number=w969, precision (6)=i16 1) -> (F-format string=w973:string)  [unwired: 2 in]
                n768 = Fract/Exp String To Number(string=w974) -> (number=w966:dbl)  [unwired: 3 in, 1 out]
                n769 = Fract/Exp String To Number(string=w975) -> (number=w964:dbl)  [unwired: 3 in, 1 out]
                n770 = Fract/Exp String To Number(string=w973) -> (number=w968:dbl)  [unwired: 3 in, 1 out]
                n771 = local write "Major Axis"(w968) -> ()
                n772 = local write "Average"(w964) -> ()
                n773 = local write "Minor Axis"(w966) -> ()
              }
            }
            n774 = case shown="\"Measrument\", Default" w878 {
              tunnel: w881 -> [w908 _]
              tunnel: w880 -> [w907 _]
              tunnel: [w904 w933] -> w879
              tunnel: w877 -> [w906 w933]
              tunnel: w876 -> [w905 _]
              tunnel: w873 -> [w903 _]
              frame "Measrument", Default {
                n775 = stacked-sequence {
                  tunnel: w908 -> [w926 _]
                  tunnel: w907 -> [w924 _]
                  tunnel: w906 -> [w922 _]
                  tunnel: w905 -> [w921 _]
                  tunnel: [w916 _] -> w904
                  tunnel: w903 -> [w909 _]
                  frame #0 {
                    n776 = call "IMAGE ANALYSIS.vi"("Enum"=POST_ANALYSIS_ENUM."SAVE IMAGE", "error in"=w922, "IMAGE FILE PATH"=w921) -> ("error out"=w920:errorcluster)  [unwired: 7 in, 1 out]
                    n777 = call "Stall Data Flow.vim"("value in"=w920, "milliseconds to wait"=u32 1000) -> ("value out"=w911:errorcluster)  [unwired: 1 out]
                    n778 = local read "Test File List :"() -> (w928:string)
                    n779 = call "IMAGE ANALYSIS.vi"("Enum"=POST_ANALYSIS_ENUM."MINIMIZE UI", "error in"=w911) -> ("error out"=w918:errorcluster)  [unwired: 8 in, 1 out]
                    n780 = Bundle By Name(cluster=T25 {"File Name"="", "Test Method"="", "Operator"="", "Fuel Description"="", "Date and time"=""} ("Main Ref"), "Test Method"=w909, "File Name"=w928) -> (w929:T25)
                    n781 = call "Stall Data Flow.vim"("value in"=w918, "milliseconds to wait"=u32 1500) -> ("value out"=w913:errorcluster)  [unwired: 1 out]
                    n782 = call "duf file read.vi"("error in (no error)"=w913, "Main Ref"=w929) -> ("error out"=w927:errorcluster, "Main Ref 2"=w925:T25)  [unwired: 8 in]
                    n783 = call "DETECTION REPORT for manual.vi"("error in (no error)"=w927, "return value 3"=w924, "Image File Path"=w926, "Main Ref"=w925) -> ("error out"=w923:errorcluster)  [unwired: 7 in]
                    n784 = call <vilib>:"Clear Errors.vi"("error in (no error)"=w923) -> ("error out"=w914:errorcluster)  [unwired: 5 in, 1 out]
                    n785 = call "IMAGE ANALYSIS.vi"("Enum"=POST_ANALYSIS_ENUM."MINIMIZE UI", "error in"=w914) -> ("error out"=w916:errorcluster)  [unwired: 8 in, 1 out]
                  }
                  frame #1 {
                    n786 = local write "Main Tab"(T2."HOME" ("Main Tab")) -> ()
                    n787 = local write "Main Dashboard Buttons"(T1."Home" ("Main Dashboard Buttons")) -> ()
                  }
                }
              }
              frame "Calibrate" {
              }
            }
          }
          frame #2 {
            n788 = Not(x=w998) -> (.not. x?=w997:bool)
            n789 = local write "Confirm Measrurement"(w997) -> ()
            n790 = local read "Calibration Tab"() -> (w996:enum32{"Measrument", "Calibrate"})
            n791 = case shown="\"Measrument\", Default" w996 {
              frame "Measrument", Default {
                (unwired) T20."HOME" ("Main Tab")
                n792 = local write "Main Tab"(T2."HOME" ("Main Tab")) -> ()
              }
              frame "Calibrate" {
              }
            }
          }
        }
      }
    }
    n793 = local read "Humidity"() -> (w741:bool)
    n794 = local read "Save Change"() -> (w746:bool)
    n795 = local read "Calibrate"() -> (w747:bool)
    n796 = local read "Auto Start Test"() -> (w742:bool)
    n797 = case shown="True" w747 {
      selector: w747 -> [_ w854]
      frame False {
      }
      frame True {
        n798 = Not(x=w854) -> (.not. x?=w853:bool)
        n799 = local write "Calibrate"(w853) -> ()
        n800 = local write "Calibration Tab"(enum32{"Measrument", "Calibrate"}."Calibrate" ("Calibration Tab")) -> ()
      }
    }
    n801 = case shown="True" w746 {
      selector: w746 -> [_ w798]
      frame False {
      }
      frame True {
        n802 = stacked-sequence {
          tunnel: w798 -> [_ _ _ _ w852]
          frame #0 {
            n803 = call "IMAGE ANALYSIS.vi"("Enum"=POST_ANALYSIS_ENUM."HIDE UI") -> ()  [unwired: 9 in, 2 out]
          }
          frame #1 {
            n804 = local read "100x gain"() -> (w800:dbl)
            n805 = local read "10x Gain"() -> (w801:dbl)
            n806 = local read "5x Gain"() -> (w802:dbl)
            n807 = Number To Fractional String(number=w801, width (-)=i16 4, precision (6)=i16 7) -> (F-format string=w823:string)  [unwired: 1 in]
            n808 = Number To Fractional String(number=0.0, width (-)=i16 4, precision (6)=i16 7) -> (F-format string=w818:string)  [unwired: 1 in]
            n809 = Number To Fractional String(number=w800, width (-)=i16 4, precision (6)=i16 7) -> (F-format string=w806:string)  [unwired: 1 in]
            n810 = Number To Fractional String(number=w802, width (-)=i16 10 ("precision (6)"), precision (6)=i16 7) -> (F-format string=w832:string)  [unwired: 1 in]
            n811 = Concatenate Strings("[CH1]" ("string"), w832, " - 5x Gain" ("string"), "\r") -> (w822:string)
            n812 = Concatenate Strings("[CH2]" ("string"), w823, " - 10x Gain" ("string"), "\r") -> (w821:string)
            n813 = Concatenate Strings("[CH3]" ("string"), w818, " - 20x Gain" ("string"), "\r") -> (w812:string)
            n814 = Concatenate Strings("[CH4]" ("string"), w806, " - 100x Gain" ("string"), "\r") -> (w805:string)
            n815 = String To Path(string="C:\\LAB-IQ\\Image Calibrate v01.dcf") -> (path=w835:path)
            n816 = Concatenate Strings(w822, w821, w812, w805) -> (w820:string)
            n817 = call <vilib>:"Write Characters To File.vi"("append to file? (new file:F)"=FALSE, "character string"=w820, "file path (dialog if empty)"=w835) -> ()  [unwired: 2 in, 1 out]
          }
          frame #2 {
            n818 = String To Path(string="C:\\LAB-IQ\\Image Calibrate v01.dcf") -> (path=w838:path)
            n819 = Open/Create/Replace File ("Open File")(file path (use dialog)=w838) -> (refnum out=w839:refnum<file>)  [unwired: 5 in, 2 out]
            n820 = for {
              N: 4 -> [_]
              tunnel: w839 -> [w845]
              i -> [w841]
              n821 = Read from Text File ("Read File")(file (use dialog)=w845) -> (text=w846:string)  [unwired: 3 in, 3 out]
              n822 = String Subset(string=w846, offset (0)=6, length (rest)=10 ("length (rest)")) -> (substring=w842:string)
              n823 = Fract/Exp String To Number(string=w842) -> (number=w840:dbl)  [unwired: 3 in, 1 out]
              n824 = case shown="3" w841 {
                tunnel: w840 -> [w847 w848 _ w849 _]
                frame 0 {
                  n825 = local write "5x Gain"(w847) -> ()
                }
                frame 1 {
                  n826 = local write "10x Gain"(w848) -> ()
                }
                frame 2 {
                }
                frame 3 {
                  n827 = local write "100x gain"(w849) -> ()
                }
                frame 4, Default {
                }
              }
            }
          }
          frame #3 {
            n828 = call "IMAGE ANALYSIS.vi"("Enum"=POST_ANALYSIS_ENUM."SHOW UI") -> ()  [unwired: 9 in, 2 out]
          }
          frame #4 {
            n829 = Not(x=w852) -> (.not. x?=w851:bool)
            n830 = local write "Save Change"(w851) -> ()
          }
        }
      }
    }
    n831 = case shown="False" w742 {
      tunnel: w741 -> [w768 _]
      frame False {
        n832 = case shown="True" w768 {
          frame False {
          }
          frame True {
            n833 = local read "Set Humidity:"() -> (w772:dbl)
            n834 = local read "Set Humidity:"() -> (w775:dbl)
            n835 = local read "Humidity ( %RH )"() -> (w776:dbl)
            n836 = Subtract(x=w772, y=2.0) -> (x-y=w770:dbl)
            n837 = Add(x=w775, y=2.0) -> (x+y=w771:dbl)
            n838 = In Range and Coerce(upper limit=w771, x=w776, lower limit=w770) -> (In Range?=w769:bool)  [unwired: 1 out]
            n839 = case shown="True" w769 {
              frame False {
              }
              frame True {
                n840 = case shown="True" "Manual Humididty Reached" {
                  selector: "Manual Humididty Reached" -> [_ w779]
                  frame False {
                  }
                  frame True {
                    n841 = Not(x=w779) -> (.not. x?=w778:bool)
                    n842 = local write "Manual Humididty Reached"(w778) -> ()
                    n843 = local read "EVENT LOG"() -> (w781:string)
                    n844 = call "Event Log.vi"("Content"="Target Humidity reached", "EVENT LOG"=w781) -> ("EVENT LOG"=w780:string)  [unwired: 8 in, 1 out]
                    n845 = local write "EVENT LOG"(w780) -> ()
                  }
                }
              }
            }
          }
        }
      }
      frame True {
        n846 = local write "Manual Humididty Reached"(TRUE ("Manual Humididty Reached")) -> ()
      }
    }
    n847 = local read "Cap Live Image"() -> (w762:bool)
    n848 = local read "SCAR MEASURMENT"() -> (w765:enum32{"Auto Scar", "Manual Scar"})
    n849 = Wait (ms)(milliseconds to wait=u32 250) -> ()  [unwired: 1 out]
    n850 = Equal?(x=w765, y=enum32{"Auto Scar", "Manual Scar"}."Manual Scar" ("SCAR MEASURMENT")) -> (x = y?=w763:bool)
    n851 = And(x=w763, y=w762) -> (x .and. y?=w761:bool)
    n852 = case shown="True" w761 {
      selector: w761 -> [_ w1077]
      frame False {
      }
      frame True {
        n853 = stacked-sequence {
          tunnel: [_ _ _ w1092 _] -> _
          tunnel: w1077 -> [_ _ _ _ w1099]
          frame #0 {
            w1078 = 0.0
            n854 = local write "Major Axis"(w1078) -> ()
            n855 = local write "Minor Axis"(w1078) -> ()
            n856 = local write "Average"(w1078) -> ()
          }
          frame #1 {
            n857 = call "CAMERA LIVE FEED FGV.vi"("Enum - Menu"=CAMERA_LIVE_FEED_ENUM."CAMERA MINIMIZE") -> ()  [unwired: 9 in, 2 out]
          }
          frame #2 {
            n858 = local read "FILE 3"() -> (w1086:string)
            n859 = call <vilib>:"Trim Whitespace.vi"("string"="C:\\LAB-IQ\\images\\") -> ("trimmed string"=w1088:string)  [unwired: 1 in]
            n860 = String To Path(string=w1088) -> (path=w1087:path)
            n861 = Concatenate Strings(w1086, ".png" ("string")) -> (w1085:string)
            n862 = Build Path(base path=w1087, name or relative path=w1085) -> (appended path=w1083:path)
            n863 = Path To String(path=w1083) -> (string=w1082:string)
            n864 = call "CAMERA LIVE FEED FGV.vi"("Enum - Menu"=CAMERA_LIVE_FEED_ENUM."CAMERA SAVE", "Image Path"=w1082) -> ("error out"=w1080:errorcluster)  [unwired: 8 in, 1 out]
            n865 = case shown="No Error" w1080 {
              frame No Error {
                n866 = One Button Dialog(message="Image saved successfully") -> ()  [unwired: 1 in, 1 out]
              }
              frame Error {
              }
            }
          }
          frame #3 {
            n867 = call "LIST FILE NAMES.vi"() -> ("error out"=w1094:errorcluster, "filenames"=w1091:string[])  [unwired: 10 in]
            n868 = call "IMAGE ANALYSIS.vi"("Enum"=POST_ANALYSIS_ENUM."SHOW UI", "error in"=w1094) -> ("error out"=w1092:errorcluster)  [unwired: 8 in, 1 out]
            n869 = property on="Test File List :" class="CmbBox"("Strings[]"=w1091) -> ()  [unwired: 2 in, 2 out]
          }
          frame #4 {
            (unwired) T24."Report" ("Main Dashboard Buttons")
            (unwired) T26."Report" ("Main Dashboard Buttons")
            n870 = Not(x=w1099) -> (.not. x?=w1098:bool)
            n871 = local write "Zoom Factore"(0.0 ("Zoom Factore")) -> ()
            n872 = local write "Cap Live Image"(w1098) -> ()
            n873 = local write "Main Tab"(T2."Adv Scar Report" ("Main Tab")) -> ()
            n874 = property on="Cap Live Image" class="Bool (strict)"("BoolText.Text"="Capture Image" ("Boolean Text.Text")) -> ()  [unwired: 2 in, 2 out]
            n875 = local write "Main Dashboard Buttons"(T1."Report" ("Main Dashboard Buttons")) -> ()
          }
        }
      }
    }
    n876 = local read "change Gain"() -> (w745:bool)
    n877 = local read "Back Square"() -> (w744:bool)
    n878 = case shown="True" w745 {
      selector: w745 -> [_ w789]
      frame False {
      }
      frame True {
        n879 = stacked-sequence {
          tunnel: w789 -> [_ w797]
          frame #0 {
            n880 = local read "Actual (µm)"() -> (w793:dbl)
            n881 = local read "Pixel Value"() -> (w792:dbl)
            n882 = local read "Magnification :"() -> (w791:string)
            n883 = Divide(x=w793, y=w792) -> (x/y=w790:dbl)
            n884 = case shown="\"10x\"" w791 {
              tunnel: w790 -> [w794 w795]
              frame "10x" {
                n885 = local write "10x Gain"(w794) -> ()
              }
              frame "5x", Default {
                n886 = local write "5x Gain"(w795) -> ()
              }
            }
          }
          frame #1 {
            n887 = Not(x=w797) -> (.not. x?=w796:bool)
            n888 = local write "change Gain"(w796) -> ()
          }
        }
      }
    }
    n889 = case shown="True" w744 {
      selector: w744 -> [_ w787]
      frame False {
      }
      frame True {
        n890 = Not(x=w787) -> (.not. x?=w786:bool)
        n891 = local write "Back Square"(w786) -> ()
        n892 = local write "Calibration Tab"(enum32{"Measrument", "Calibrate"}."Measrument" ("Calibration Tab")) -> ()
      }
    }
    n893 = local read "Rectangle Tool"() -> (w756:bool)
    n894 = local read "Clear ROI Tool"() -> (w755:bool)
    n895 = local read "Open Image"() -> (w760:bool)
    n896 = local read "line tool"() -> (w757:bool)
    n897 = local read "OUT"() -> (w758:bool)
    n898 = local read "In"() -> (w759:bool)
    n899 = case shown="True" w760 {
      selector: w760 -> [_ w1065]
      tunnel: [w1061 w1067] -> _
      tunnel: w750 -> [w1061 w1066]
      frame False {
      }
      frame True {
        n900 = Not(x=w1065) -> (.not. x?=w1064:bool)
        n901 = local write "Open Image"(w1064) -> ()
        n902 = call "IMAGE ANALYSIS.vi"("Enum"=POST_ANALYSIS_ENUM."HIDE UI", "error in"=w1066) -> ("error out"=w1074:errorcluster)  [unwired: 8 in, 1 out]
        n903 = call "File Dialog"("start path"=path "C:/LAB-IQ/images", "error in"=w1074) -> ("selected path"=w1063:path, "error out"=w1072:errorcluster)  [unwired: 10 in, 2 out]
        "Image path  2" <- w1063
        n904 = call <vilib>:"Clear Errors.vi"("error in (no error)"=w1072) -> ("error out"=w1071:errorcluster)  [unwired: 5 in, 1 out]
        n905 = call "IMAGE ANALYSIS.vi"("Enum"=POST_ANALYSIS_ENUM."OPEN FILE", "error in"=w1071, "File Path"=w1063) -> ("error out"=w1070:errorcluster)  [unwired: 7 in, 1 out]
